vi "Determine Warnings 4.vi"() -> ()   [LabVIEW 2014]
panel:
  in  "Current Wind Speed":dbl
  in  "Max Wind Speed":dbl
  out "Warning?":bool
  out "Warning Text":string
  in  "Max Temp":dbl
  in  "Min Temp":dbl
  in  "Current Temp":dbl
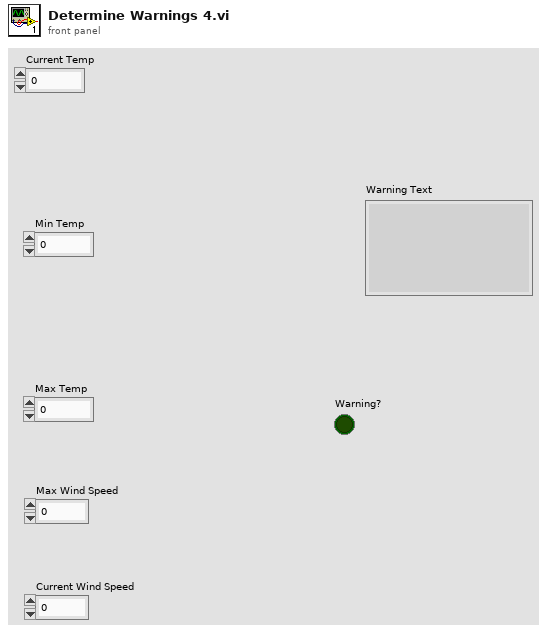
[diagram p1: front panel]
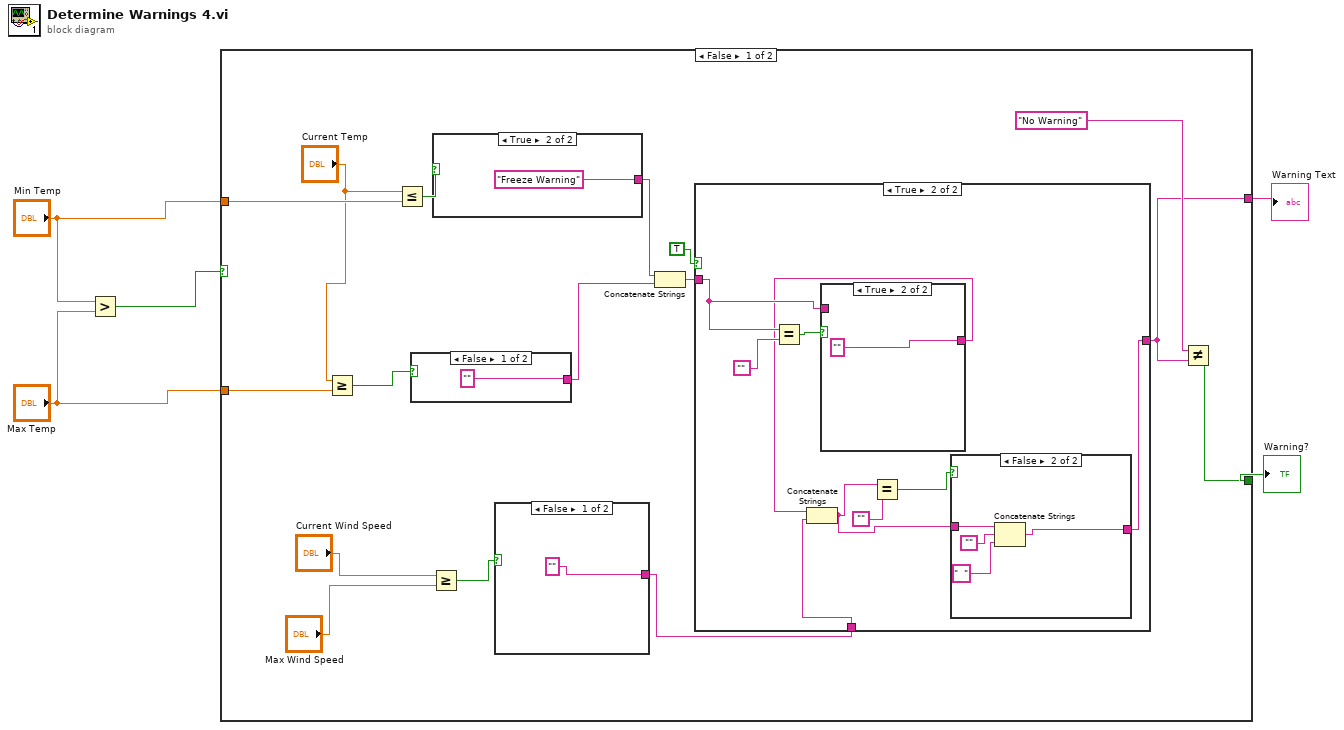
[diagram p0: block diagram]
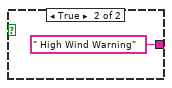
[diagram p2: hidden frame]
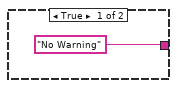
[diagram p4: hidden frame]
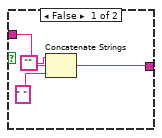
[diagram p5: hidden frame]
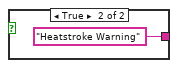
[diagram p6: hidden frame]
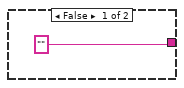
[diagram p7: hidden frame]
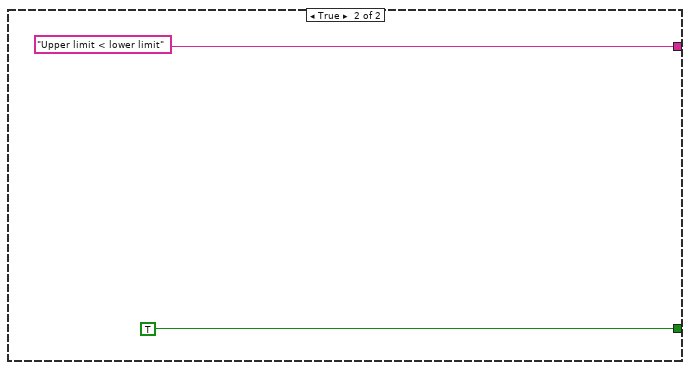
[diagram p8: hidden frame]
diagram:
  n1 = Greater?(x="Min Temp", y="Max Temp") -> (0:w2:bool)
  n2 = case shown="False" w2 {
    tunnel: "Min Temp" -> [w21 _]
    tunnel: "Max Temp" -> [w20 _]
    tunnel: [w11 "Upper limit < lower limit"] -> w5
    tunnel: [w10 TRUE ("Warning?")] -> w1
    frame False {
      n3 = Greater Or Equal?(x="Current Temp", y=w20) -> (x >= y?=w17:bool)
      n4 = Less Or Equal?(x="Current Temp", y=w21) -> (x <= y?=w18:bool)
      n5 = case shown="False" w17 {
        tunnel: ["" "Heatstroke Warning"] -> w14
        frame False {
        }
        frame True {
        }
      }
      n6 = Greater Or Equal?(x="Current Wind Speed", y="Max Wind Speed") -> (x >= y?=w7:bool)
      n7 = case shown="True" w18 {
        tunnel: ["" "Freeze Warning"] -> w15
        frame False {
        }
        frame True {
        }
      }
      n8 = case shown="False" w7 {
        tunnel: ["" " High Wind Warning"] -> w6
        frame False {
        }
        frame True {
        }
      }
      n9 = Concatenate Strings(w15, w14) -> (w16:string)
      n10 = case shown="True" TRUE {
        tunnel: w16 -> [w24 w31]
        tunnel: [w24 w25] -> w11
        tunnel: w6 -> [_ w29]
        frame False {
        }
        frame True {
          n11 = Equal?(x=w31, y="") -> (x = y?=w32:bool)
          n12 = case shown="True" w32 {
            tunnel: w31 -> [w41 _]
            tunnel: [w39 ""] -> w28
            frame False {
              n13 = Concatenate Strings("", w41, " ") -> (w39:string)
            }
            frame True {
            }
          }
          n14 = Concatenate Strings(w28, w29) -> (w26:string)
          n15 = Equal?(x=w26, y="") -> (x = y?=w30:bool)
          n16 = case shown="False" w30 {
            tunnel: w26 -> [_ w36]
            tunnel: ["No Warning" w35] -> w25
            frame True {
            }
            frame False {
              n17 = Concatenate Strings(w36, "", "  ") -> (w35:string)
            }
          }
        }
      }
      n18 = Not Equal?(x="No Warning", y=w11) -> (x != y?=w10:bool)
    }
    frame True {
    }
  }
  "Warning Text" <- w5
  "Warning?" <- w1
